vi "IC_VCDInterfaces.vi"(1 "Interface":u16(ring) items=["Range", "Switch", "Button", "Mapstrings", "Absolute Values"], 2 "Element ID":u16(ring) items=["Value", "Auto", "One Push", "Whitebalance Bue", "Whitebalance Red", "Auto Reference", "Trigger Polarity", "Trigger Mode", "Reset Value", "GP IO Input", "GP IO Output", "GP IO Write", "GP IO Read", "Strope Polarity", "Strobe Duration", "Strobe Delay"], 3 "Property":u16(ring) items=["Brightness", "Contrast", "Hue", "Saturation", "Sharpness", "Gamma", "Color Enable", "White Balance", "Backlight Compensation", "Gain", "Pan", "Tilt", "Roll", "Zoom", "Exposure", "Iris", "Focus", "Trigger Mode", "VCR Compatibility", "Signal Detected", "Testpattern", "GP IO", "Strobe"]) -> (0 "Interface Path":string)   [LabVIEW 2020]
doc: "This VI creates the VCD Interface in order to access a VCD property"
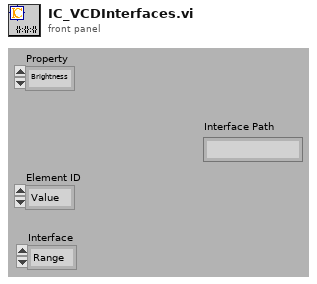
[diagram p1: front panel]
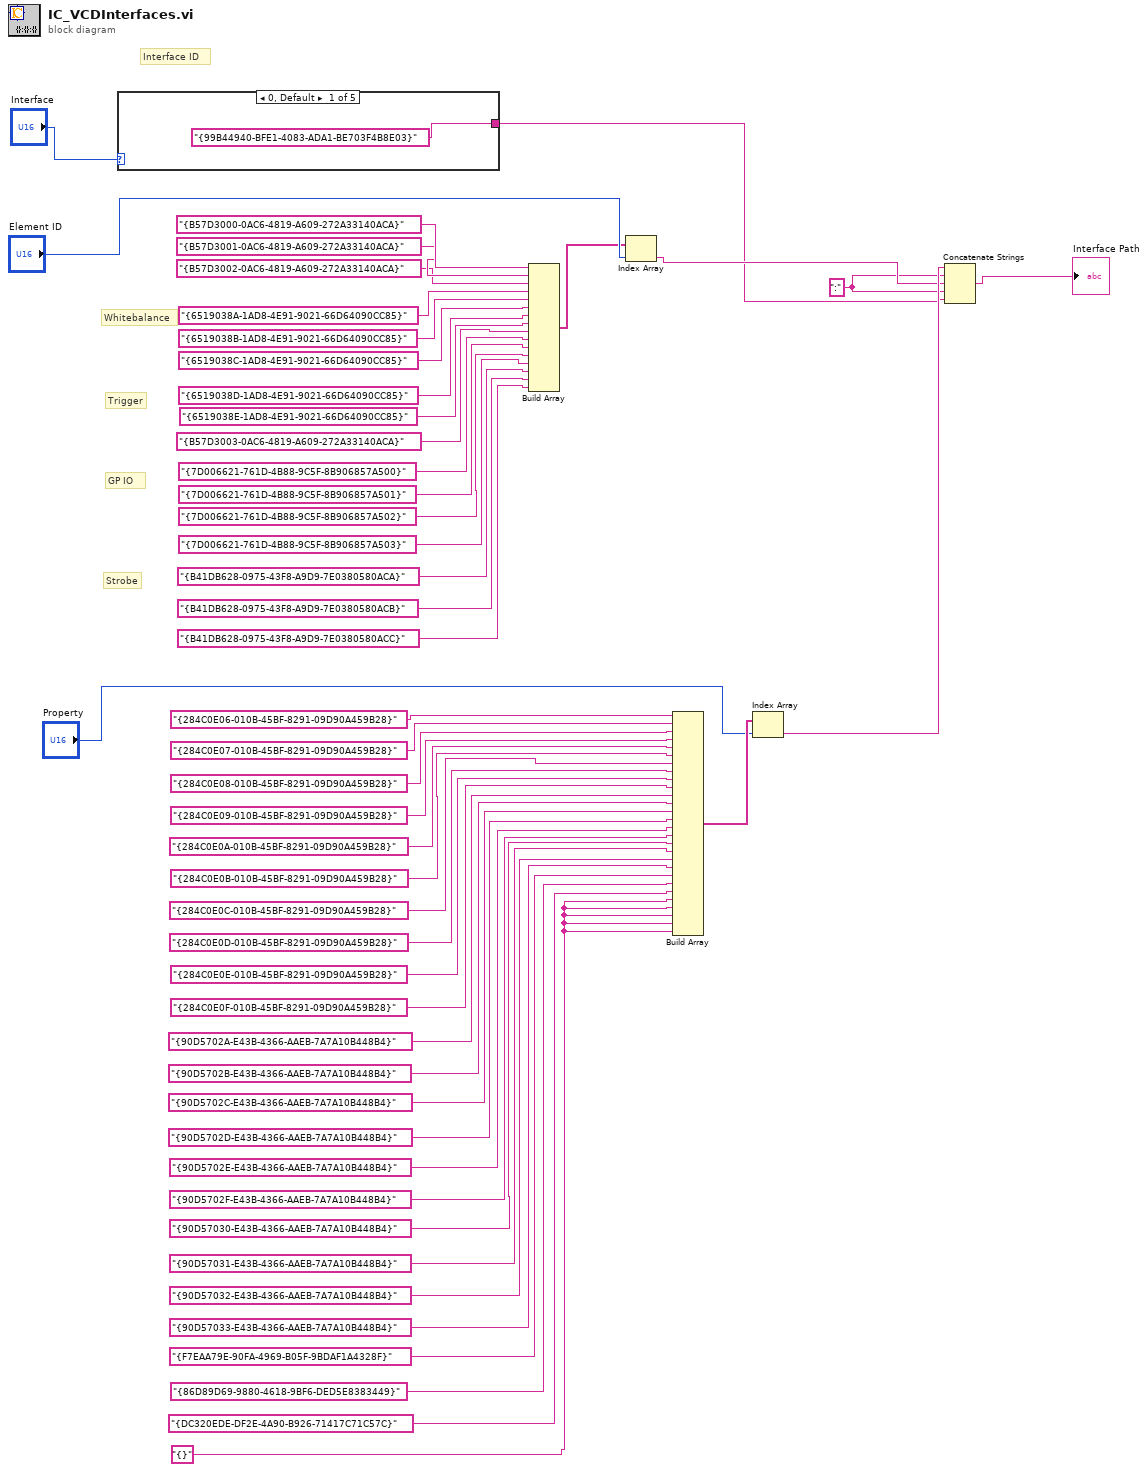
[diagram p0: block diagram]
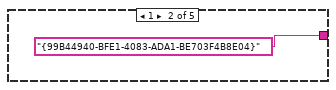
[diagram p2: hidden frame]
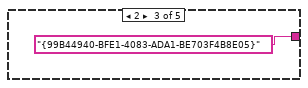
[diagram p3: hidden frame]
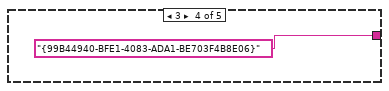
[diagram p4: hidden frame]
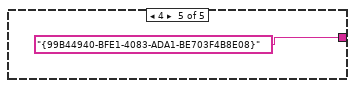
[diagram p5: hidden frame]
diagram:
  w3 = ":"
  w6 = "{}"
  # "Strobe"
  # "Whitebalance"
  # "Trigger"
  # "GP IO"
  # "Interface ID"
  n1 = case shown="0, Default" "Interface" {
    tunnel: ["{99B44940-BFE1-4083-ADA1-BE703F4B8E03}" "{99B44940-BFE1-4083-ADA1-BE703F4B8E04}" "{99B44940-BFE1-4083-ADA1-BE703F4B8E05}" "{99B44940-BFE1-4083-ADA1-BE703F4B8E06}" "{99B44940-BFE1-4083-ADA1-BE703F4B8E08}"] -> w2
    frame 0, Default {
    }
    frame 1 {
    }
    frame 2 {
    }
    frame 3 {
    }
    frame 4 {
    }
  }
  n2 = Build Array("{B57D3000-0AC6-4819-A609-272A33140ACA}", "{B57D3001-0AC6-4819-A609-272A33140ACA}", "{B57D3002-0AC6-4819-A609-272A33140ACA}", "{6519038A-1AD8-4E91-9021-66D64090CC85}", "{6519038B-1AD8-4E91-9021-66D64090CC85}", "{6519038C-1AD8-4E91-9021-66D64090CC85}", "{6519038D-1AD8-4E91-9021-66D64090CC85}", "{6519038E-1AD8-4E91-9021-66D64090CC85}", "{B57D3003-0AC6-4819-A609-272A33140ACA}", "{7D006621-761D-4B88-9C5F-8B906857A500}", "{7D006621-761D-4B88-9C5F-8B906857A501}", "{7D006621-761D-4B88-9C5F-8B906857A502}", "{7D006621-761D-4B88-9C5F-8B906857A503}", "{B41DB628-0975-43F8-A9D9-7E0380580ACA}", "{B41DB628-0975-43F8-A9D9-7E0380580ACB}", "{B41DB628-0975-43F8-A9D9-7E0380580ACC}") -> (w48:string[])
  n3 = Index Array(array=w48, index="Element ID") -> (element=w4:string)
  n4 = Build Array("{284C0E06-010B-45BF-8291-09D90A459B28}", "{284C0E07-010B-45BF-8291-09D90A459B28}", "{284C0E08-010B-45BF-8291-09D90A459B28}", "{284C0E09-010B-45BF-8291-09D90A459B28}", "{284C0E0A-010B-45BF-8291-09D90A459B28}", "{284C0E0B-010B-45BF-8291-09D90A459B28}", "{284C0E0C-010B-45BF-8291-09D90A459B28}", "{284C0E0D-010B-45BF-8291-09D90A459B28}", "{284C0E0E-010B-45BF-8291-09D90A459B28}", "{284C0E0F-010B-45BF-8291-09D90A459B28}", "{90D5702A-E43B-4366-AAEB-7A7A10B448B4}", "{90D5702B-E43B-4366-AAEB-7A7A10B448B4}", "{90D5702C-E43B-4366-AAEB-7A7A10B448B4}", "{90D5702D-E43B-4366-AAEB-7A7A10B448B4}", "{90D5702E-E43B-4366-AAEB-7A7A10B448B4}", "{90D5702F-E43B-4366-AAEB-7A7A10B448B4}", "{90D57030-E43B-4366-AAEB-7A7A10B448B4}", "{90D57031-E43B-4366-AAEB-7A7A10B448B4}", "{90D57032-E43B-4366-AAEB-7A7A10B448B4}", "{90D57033-E43B-4366-AAEB-7A7A10B448B4}", "{F7EAA79E-90FA-4969-B05F-9BDAF1A4328F}", "{86D89D69-9880-4618-9BF6-DED5E8383449}", "{DC320EDE-DF2E-4A90-B926-71417C71C57C}", w6, w6, w6, w6, w6) -> (w8:string[])
  n5 = Index Array(array=w8, index="Property") -> (element=w5:string)
  n6 = Concatenate Strings(w5, w3, w4, w3, w2) -> (→"Interface Path":string)
